vi "SDCP - Standard Message Frames FGV.vi"(4 "Frame priority in":bool, 5 "error in (no error)":errorcluster, 6 "Command":T1, 7 "FID":i32, 8 "SMF in":u8[](array[numeric])) -> (0 "error out":errorcluster, 2 "Frame priority out":bool, 3 "SMF out":u8[](array[numeric]))   [LabVIEW 2020]
uses:
  Typedefs/SDCP - Standard Message Frames FGV - Commands.ctl
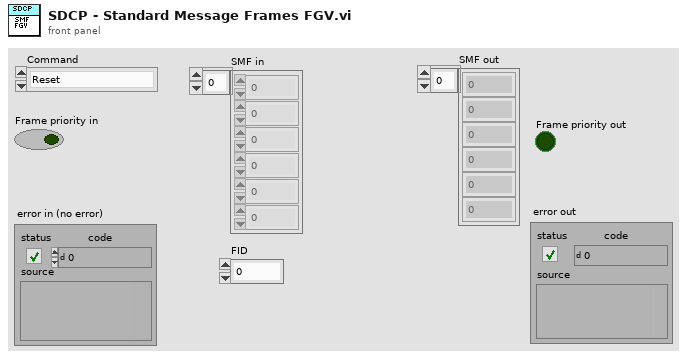
[diagram p1: front panel]
types:
  T1 = typedef "SDCP - Standard Message Frames FGV - Commands.ctl" = enum16{"Reset", "Read", "Write", "Set Priority"}
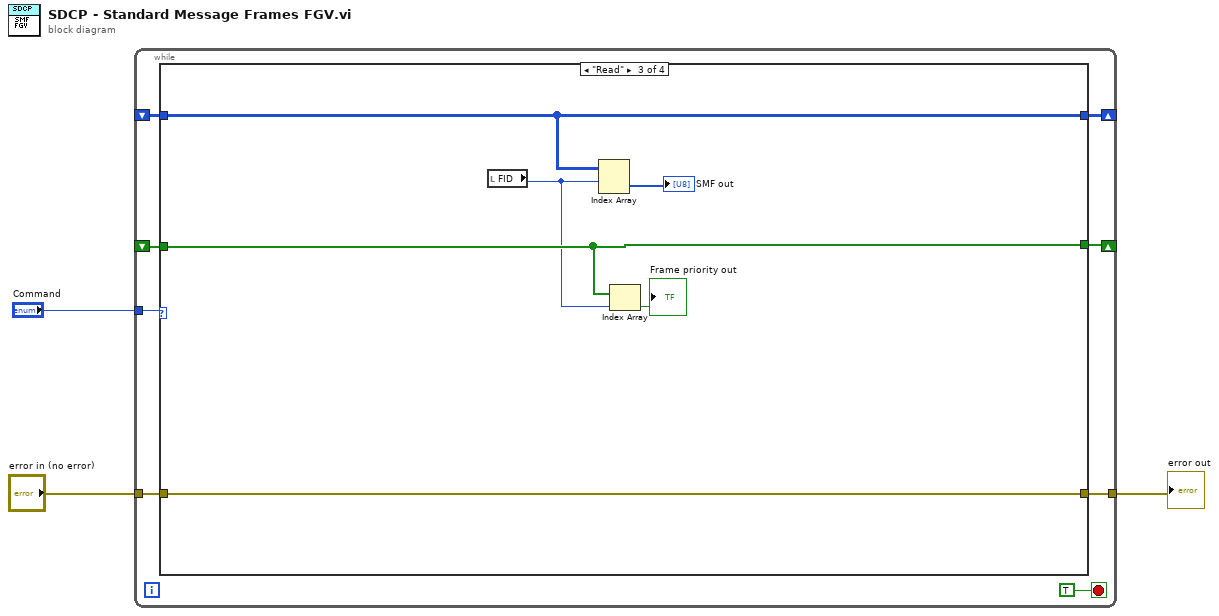
[diagram p0: block diagram]
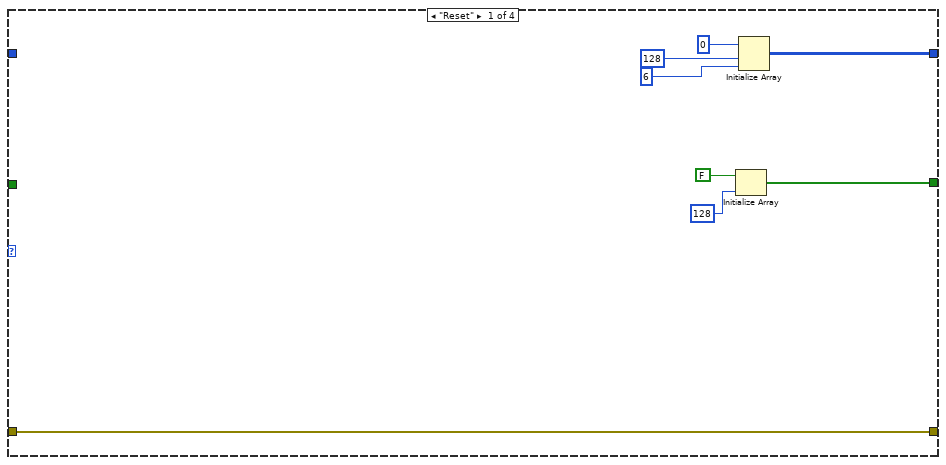
[diagram p2: hidden frame]
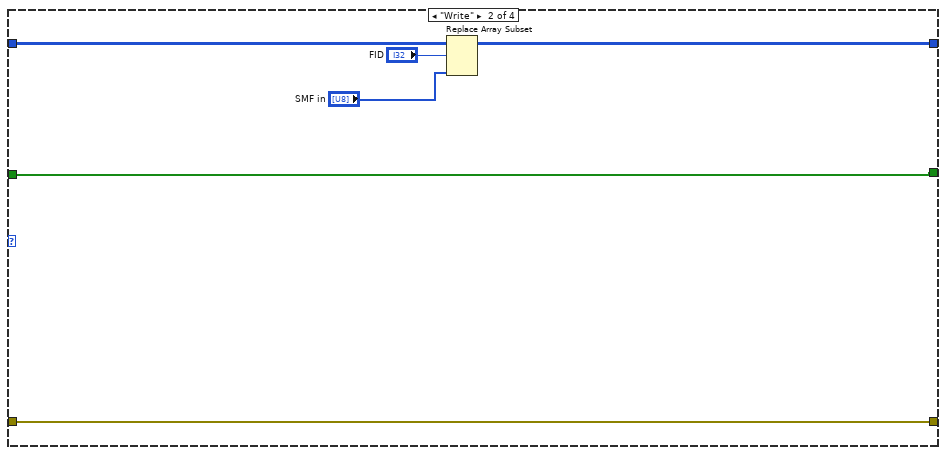
[diagram p3: hidden frame]
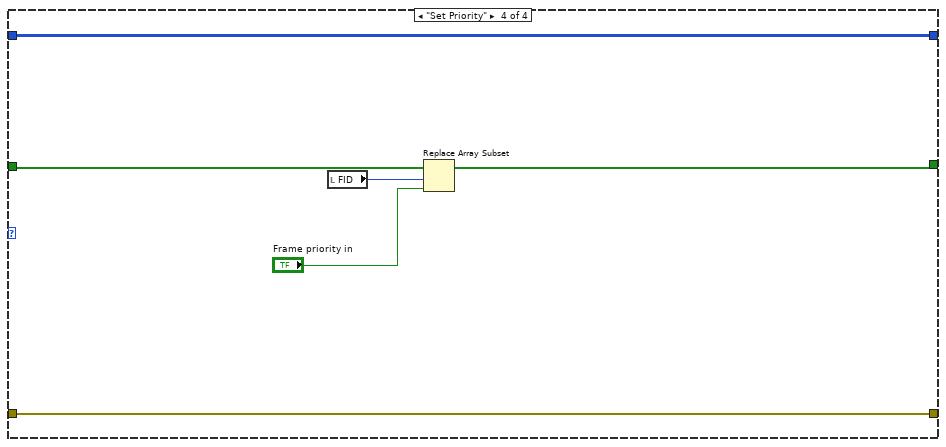
[diagram p4: hidden frame]
diagram:
  n1 = while {
    tunnel: "error in (no error)" -> [w10]
    tunnel: "Command" -> [w9]
    tunnel: [w8] -> w1
    shift-right: [w7] -> _
    shift-left: _ -> [w6]
    shift-right: [w5] -> _
    shift-left: _ -> [w4]
    stop <- TRUE stop-if-true
    n2 = case shown="\"Read\"" w9 {
      tunnel: w10 -> [w19 w21 w29 w33]
      tunnel: [w19 w21 w29 w33] -> w8
      tunnel: [w15 w24 w31 w37] -> w7
      tunnel: w6 -> [_ w25 w31 w37]
      tunnel: [w12 w20 w28 w32] -> w5
      tunnel: w4 -> [_ w20 w28 w36]
      frame "Reset" {
        n3 = Initialize Array(FALSE, 128 ("dimension size")) -> (w12:bool[])
        n4 = Initialize Array(u8 0, 128, 6) -> (w15:u8[][])
      }
      frame "Write" {
        n5 = Replace Array Subset(array=w25, new element="SMF in", index (row)="FID") -> (w24:u8[][])  [unwired: 1 in]
      }
      frame "Read" {
        n6 = local read "FID"() -> (w27:i32)
        n7 = Index Array(array=w31, index (row)=w27) -> (element=→"SMF out":u8[])  [unwired: 1 in]
        n8 = Index Array(array=w28, index=w27) -> (element=→"Frame priority out":bool)
      }
      frame "Set Priority" {
        n9 = local read "FID"() -> (w35:i32)
        n10 = Replace Array Subset(array=w36, new element="Frame priority in", index=w35) -> (w32:bool[])
      }
    }
  }
  "error out" <- w1
